vi "Parse String.vi"(7 "Channel Direction":string, 8 "error in (no error)":errorcluster, 11 "Read String":string) -> (0 "error out":errorcluster, 1 "DataTypes":T1[](array[typedef]), 2 "URLs":string[](array[string]), 3 "Name":string[](array[string]))   [LabVIEW 2017, in "TXT.lvlib" / "TXT.lvclass"]
uses:
  TXT.lvclass
  <vilib>/Utility/Data Type/Type Definitions/Data Type.ctl
  TXT Global.vi
  <vilib>/Utility/error.llb/Error Cluster From Error Code.vi
  <vilib>/ErrorRing/Error Ring.xnode
  <vilib>/Utility/Data Type/NI_Data Type.lvlib
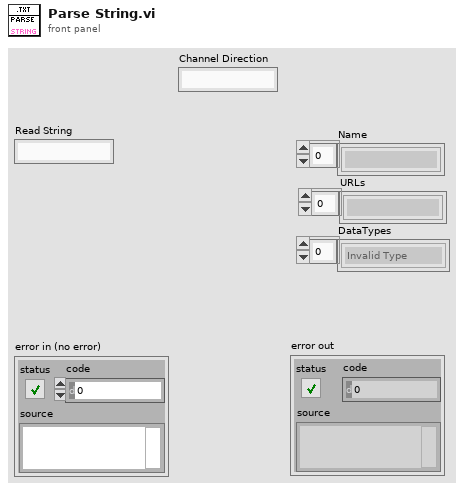
[diagram p1: front panel]
types:
  T1 = typedef "NI_Data Type.lvlib/Data Type.ctl" = enum8{"Invalid Type", "Void", "I8", "I16", "I32", "I64", "U8", "U16", "U32", "U64", "Single Float", "Double Float", "Extended Float", "Single Complex", "Double Complex", "Extended Complex", "Enum U8", "Enum U16", "Enum U32", "Enum U64", "Single Float With Unit", "Double Float With Unit", "Extended Float With Unit", "Single Complex with Unit", "Double Complex with Unit", "Extended Complex with Unit", "Boolean", "String", "Path", "Picture", "Tag", "Array", "Cluster", "Variant", "LV Variant", "Waveform", "Timestamp", "Digital Waveform", "Digital Data", "ExpressData", "Refnum", "External Data", "VI", "Poly VI", "LabVIEW Class Instance", "Fixed Point"}
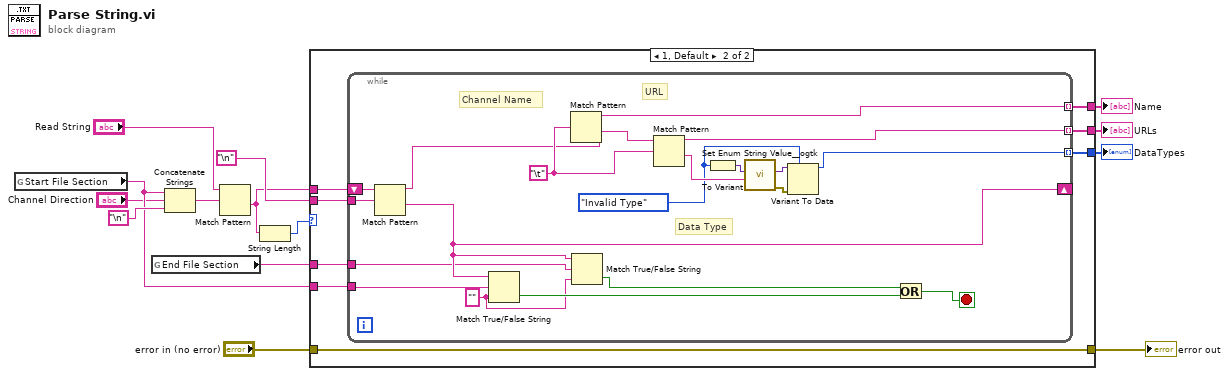
[diagram p0: block diagram]
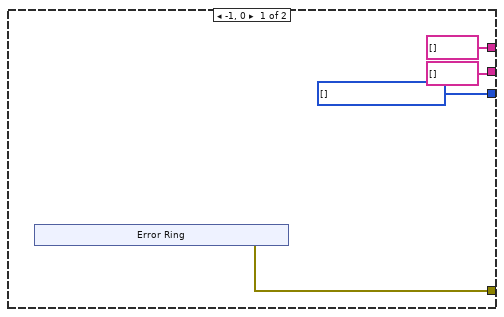
[diagram p2: hidden frame]
diagram:
  n1 = global read "TXT Global.vi" "Start File Section"() -> (w11:string)
  n2 = global read "TXT Global.vi" "End File Section"() -> (w6:string)
  n3 = Concatenate Strings(w11, "Channel Direction", "\n") -> (w14:string)
  n4 = Match Pattern(string="Read String", regular expression=w14) -> (after substring=w2:string)  [unwired: 1 in, 3 out]
  n5 = String Length(string=w2) -> (length=w1:i32)
  n6 = case shown="1, Default" w1 {
    tunnel: w2 -> [_ w31]
    tunnel: "\n" -> [_ w30]
    tunnel: w11 -> [_ w29]
    tunnel: [string[] [] w28] -> w10
    tunnel: [string[] [] w27] -> w9
    tunnel: w6 -> [_ w26]
    tunnel: [w16 w25] -> w5
    tunnel: "error in (no error)" -> [_ w24]
    tunnel: [w15 w24] -> w3
    frame -1, 0 {
      w16 = T1[] [] items=["Invalid Type", "Void", "I8", "I16", "I32", "I64", "U8", "U16", "U32", "U64", "Single Float", "Double Float", "Extended Float", "Single Complex", "Double Complex", "Extended Complex", "Enum U8", "Enum U16", "Enum U32", "Enum U64", "Single Float With Unit", "Double Float With Unit", "Extended Float With Unit", "Single Complex with Unit", "Double Complex with Unit", "Extended Complex with Unit", "Boolean", "String", "Path", "Picture", "Tag", "Array", "Cluster", "Variant", "LV Variant", "Waveform", "Timestamp", "Digital Waveform", "Digital Data", "ExpressData", "Refnum", "External Data", "VI", "Poly VI", "LabVIEW Class Instance", "Fixed Point"]
      n7 = xnode "Error Ring"() -> ("error out"=w15:errorcluster)
    }
    frame 1, Default {
      n8 = while {
        tunnel: w30 -> [w51]
        tunnel: w29 -> [w50]
        tunnel: [w47] -> w28 mode=indexing
        tunnel: [w45] -> w27 mode=indexing
        shift-right: [w41] -> _
        shift-left: w31 -> [w43]
        tunnel: w26 -> [w38]
        tunnel: [w32] -> w25 mode=indexing
        stop <- w42 stop-if-true
        w33 = Data_Type."Invalid Type" ("Type")
        w46 = "\t"
        w40 = "" ("false string")
        # "Data Type"
        # "URL"
        # "Channel Name"
        n9 = Match Pattern(string=w43, regular expression=w51) -> (before substring=w44:string, after substring=w41:string)  [unwired: 1 in, 2 out]
        n10 = Match True/False String(2:w40, 3:w50, 4:w41) -> (0:w49:bool)  [unwired: 1 out]
        n11 = Match Pattern(string=w44, regular expression=w46) -> (before substring=w47:string, after substring=w48:string)  [unwired: 1 in, 2 out]
        n12 = Match True/False String(2:w40, 3:w38, 4:w41) -> (0:w39:bool)  [unwired: 1 out]
        n13 = Match Pattern(string=w48, regular expression=w46) -> (before substring=w45:string, after substring=w37:string)  [unwired: 1 in, 2 out]
        n14 = To Variant(anything=w33) -> (Variant=w36:variant)
        n15 = call <userlib>:"Set Enum String Value__ogtk.vi"("String Value"=w37, "Default Enum Value"=w36) -> ("error out"=w35:errorcluster, "Enum"=w34:variant)  [unwired: 8 in]
        n16 = Variant To Data(error in=w35, type=w33, Variant=w34) -> (data=w32:T1)  [unwired: 1 out]
        n17 = Or(x=w39, y=w49) -> (x .or. y?=w42:bool)
      }
    }
  }
  "Name" <- w10
  "URLs" <- w9
  "DataTypes" <- w5
  "error out" <- w3
